vi "Initialize Sink.vi"(11 "Log Sink in":refnum<class "Log Sink.lvclass">) -> (0 "error out":errorcluster, 3 "Log Sink out":refnum<class "Log Sink.lvclass">)   [LabVIEW 2020, in "Composed Log.lvlib" / "Log Sink.lvclass"]
uses:
  <vilib>/gpm_packages/@cs/event-logger/Source/Composed Log/Log Sink/Log Sink.lvclass
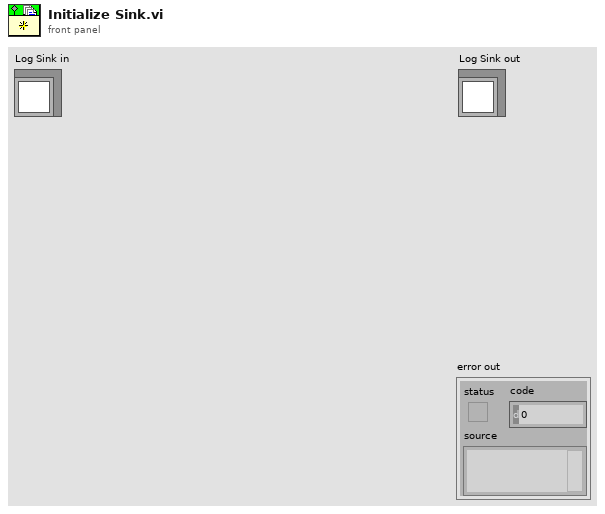
[diagram p1: front panel]
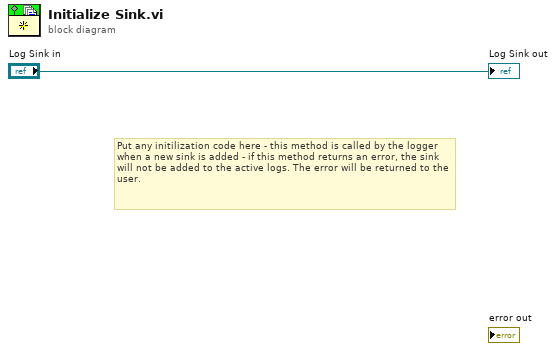
[diagram p0: block diagram]
diagram:
  # "Put any initilization code here - this method is called by the logger when a new sink is added - if this method returns an error, the sink will not be added to the active logs. The error will be returned to the user."
  "Log Sink out" <- "Log Sink in"
